vi "Test Type Conversion.vi"() -> ()   [LabVIEW 2020, in "CDM-Config.lvlib"]
uses:
  CDM-Config.lvlib
  Config Manager/Config Manager.lvclass/Config Manager.ctl
  Config Element/Set Owner.vi
  Config Element/Write Variant Value.vi
  Config Element/Config Element.lvclass
  Config Manager/Config Manager.lvclass
panel:
  out "U16 Value 2":u16
  out "error out":errorcluster
  out "U16 Value":u16
  out "String Value":string
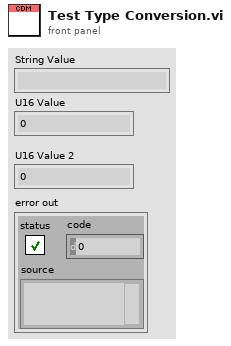
[diagram p1: front panel]
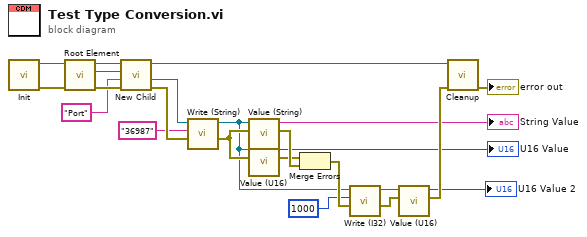
[diagram p0: block diagram]
diagram:
  n1 = call "Init.vi"() -> ("error out"=w15:errorcluster, "Config Manager out"=w18:refnum<class "Config Manager.lvclass">)  [unwired: 10 in]
  n2 = call "Root Element.vi"("error in (no error)"=w15, "Config Manager in"=w18) -> ("error out"=w14:errorcluster, "Root Element"=w16:refnum<class "Config Element.lvclass">, "Config Manager out"=w17:refnum<class "Config Manager.lvclass">)  [unwired: 7 in]
  n3 = call "New Child.vi"("error in (no error)"=w14, "Child Name"="Port", "Parent"=w16, "Config Manager in"=w17) -> ("error out"=w19:errorcluster, "New Child"=w12:refnum<class "Config Element.lvclass">, "Config Manager out"=w7:refnum<class "Config Manager.lvclass">)  [unwired: 5 in]
  n4 = call "Write (String).vi"("error in (no error)"=w19, "String Value"="36987", "Config Element in"=w12) -> ("error out"=w20:errorcluster, "Config Element out"=w5:refnum<class "Config Element.lvclass">)  [unwired: 7 in]
  n5 = call "Value (String).vi"("error in (no error)"=w20, "Config Element in"=w5) -> ("error out"=w21:errorcluster, "String Value"=→"String Value":string)  [unwired: 8 in]
  n6 = call "Value (U16).vi"("error in (no error)"=w20, "Config Element in"=w5) -> ("error out"=w8:errorcluster, "U16 Value"=→"U16 Value":u16)  [unwired: 8 in]
  n7 = Merge Errors(w8, w21) -> (w22:errorcluster)
  n8 = call "Write (I32).vi"("error in (no error)"=w22, "I32 Value"=1000, "Config Element in"=w5) -> ("error out"=w2:errorcluster, "Config Element out"=w3:refnum<class "Config Element.lvclass">)  [unwired: 7 in]
  n9 = call "Value (U16).vi"("error in (no error)"=w2, "Config Element in"=w3) -> ("error out"=w23:errorcluster, "U16 Value"=→"U16 Value 2":u16)  [unwired: 8 in]
  n10 = call "Cleanup.vi"("error in (no error)"=w23, "Config Manager in"=w7) -> ("error out"=→"error out":errorcluster)  [unwired: 9 in]
